vi "Begin.vi"   [LabVIEW 2013]
uses:
  <vilib>/Rock Robotics/SystemInterfaces/DIO/FPGA_DIOPWMChannel.ctl
  <vilib>/Rock Robotics/WPI/SafetyOutput/WPI_SafetyOutputConfigMenu.ctl
  <vilib>/Rock Robotics/SystemInterfaces/DIO/FPGA_DIOChannel.ctl
  <vilib>/Rock Robotics/SystemInterfaces/AI/FPGA_AIGyroChannel.ctl
  <vilib>/Rock Robotics/SystemInterfaces/Typedef/FPGA_TypedefDigitalModule.ctl
  <vilib>/Rock Robotics/WPI/RobotDrive/WPI_RobotDriveOpen4MotorWithJaguar.vi
  <vilib>/Rock Robotics/WPI/Counter/WPI_CounterDigitalInputToDigitalSource.vi
  <vilib>/Rock Robotics/WPI/Counter/WPI_CounterOpen Semi Period Mode.vi
types:
  T1 = typedef "FPGA_DIOChannel.ctl" = enum8{"DIO 1", "DIO 2", "DIO 3", "DIO 4", "DIO 5", "DIO 6", "DIO 7", "DIO 8", "DIO 9", "DIO 10", "DIO 11", "DIO 12", "DIO 13", "DIO 14", "Invalid"}
  T2 = typedef "FPGA_TypedefDigitalModule.ctl" = enum16{"Digital Module 1", "Digital Module 2"}
  T3 = typedef "FPGA_AIGyroChannel.ctl" = enum8{"AI 1", "AI 2", "Invalid"}
  T4 = typedef "WPI_SafetyOutputConfigMenu.ctl" = enum16{"Enable", "Disable"}
  T5 = typedef "FPGA_DIOPWMChannel.ctl" = enum8{"PWM 1", "PWM 2", "PWM 3", "PWM 4", "PWM 5", "PWM 6", "PWM 7", "PWM 8", "PWM 9", "PWM 10", "Invalid"}
  T6 = typedef "WPI_DigitalInputDevRef.ctl" = cluster{"DevStatus":errorcluster, "DIO Channel":T1, "Digital Module":T2}
  T7 = typedef "WPI_RobotDriveDevRef.ctl" = cluster{"DevStatus":errorcluster, "Motors[]":T8[], "Square Inputs":bool, "Max Output":dbl, "Isochronous":bool}
  T8 = typedef "WPI_MotorControlDeviceRef.ctl" = cluster{"DeviceStatus":errorcluster, "Type":enum16{"PWM", "CAN"}, "PWM":cluster{"Digital Module":T2, "PWM Channel":T5, "DeadBand":T9}, "CAN":cluster{"Device Number":u8, "Control Mode":T10, "Semaphore":T11, "Max Vout":dbl}, "Invert":bool, "TransformRef":T12, "InvTransformRef":T12}
  T9 = typedef "WPI_PWMDeadband.ctl" = cluster{"Name":string, "maxPositivePwm":i32, "minPositivePwm":i32, "centerPwm":i32, "maxNegativePwm":i32, "minNegativePwm":i32, "angularRange":u16}
  T10 = typedef "WPI_CANJaguar_ControlMode.ctl" = enum8{"Percent VBus", "Current", "Speed", "Position", "Voltage"}
  T11 = typedef "Semaphore RefNum" = refnum<k1>
  T12 = typedef "WPI_PWMTransform_ConPane.ctl" = refnum<vi>
  T13 = typedef "FPGA_CounterEncoderSourceConvertionLVSourceType.ctl" = cluster{"DevStatus":errorcluster, "AnalogTriggerMode?":bool, "DigitalMode":cluster{"Digital Module":T2, "DIO Channel":T14}, "AnalogTriggerMode":cluster{"AnalogTriggerIndex":T15, "OutputType":T16}}
  T14 = typedef "FPGA_DIODigitalSourceChannel.ctl" = enum8{"DIO 1", "DIO 2", "DIO 3", "DIO 4", "DIO 5", "DIO 6", "DIO 7", "DIO 8", "DIO 9", "DIO 10", "DIO 11", "DIO 12", "DIO 13", "DIO 14", "Disabled"}
  T15 = typedef "FPGA_AnalogTriggerIndex.ctl" = enum8{"Trig 0", "Trig 1", "Trig 2", "Trig 3", "Trig 4", "Trig 5", "Trig 6", "Trig 7", "Invalid"}
  T16 = typedef "FPGA_AnalogTriggerOutType.ctl" = enum16{"InWindow", "TriggerState", "Rising", "Falling"}
  T17 = typedef "WPI_EncoderDevRef.ctl" = cluster{"DevStatus":errorcluster, "EncoderIndex":T18, "CounterIndex":T19, "DistancePerCount":dbl, "Decoding Type":T20}
  T18 = typedef "FPGA_EncoderIdx.ctl" = enum8{"Enc 0", "Enc 1", "Enc 2", "Enc 3", "Invalid"}
  T19 = typedef "FPGA_CounterCtrSystemIndex.ctl" = enum8{"Ctr 0", "Ctr 1", "Ctr 2", "Ctr 3", "Ctr 4", "Ctr 5", "Ctr 6", "Ctr 7", "Invalid"}
  T20 = typedef "WPI_EncoderType.ctl" = enum16{"1x", "2x", "4x"}
  T21 = typedef "WPI_GyroDevRef.ctl" = cluster{"DevStatus":errorcluster, "Analog Module":T22, "Analog Channel":T23, "Offset":dbl, "Gain (VoltsPerDegree/Second)":dbl}
  T22 = typedef "FPGA_TypedefAnalogModule.ctl" = enum16{"Analog Module 1", "Analog Module 2"}
  T23 = typedef "FPGA_AIChannel.ctl" = enum8{"AI 1", "AI 2", "AI 3", "AI 4", "AI 5", "AI 6", "AI 7", "AI 8", "Invalid"}
  T24 = typedef "WPI_CounterDevRef.ctl" = cluster{"DevStatus":errorcluster, "CntIndex":T19}
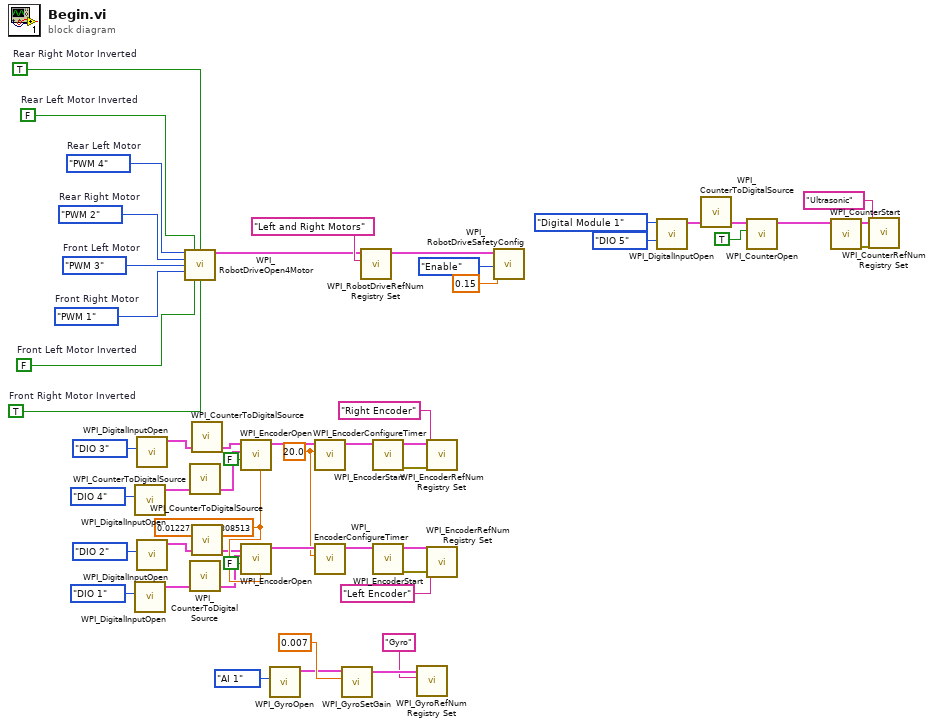
[diagram p0: block diagram]
diagram:
  w44 = 0.01227184630308513 ("DistancePerCount")
  w16 = 20.0 ("Minimum Rate")
  w8 = TRUE  # Front Right Motor Inverted
  w7 = FALSE  # Front Left Motor Inverted
  w6 = TRUE  # Rear Right Motor Inverted
  w5 = FALSE  # Rear Left Motor Inverted
  w4 = FPGA_DIOPWMChannel."PWM 1"  # Front Right Motor
  w3 = FPGA_DIOPWMChannel."PWM 3"  # Front Left Motor
  w2 = FPGA_DIOPWMChannel."PWM 2"  # Rear Right Motor
  w1 = FPGA_DIOPWMChannel."PWM 4"  # Rear Left Motor
  n1 = call <vilib>:"WPI_DigitalInputOpen.vi"("DIO Channel"=FPGA_DIOChannel."DIO 4") -> ("DigitalInputDevRef"=w33:T6)  [unwired: 9 in, 1 out]
  n2 = call <vilib>:"WPI_DigitalInputOpen.vi"("DIO Channel"=FPGA_DIOChannel."DIO 1") -> ("DigitalInputDevRef"=w19:T6)  [unwired: 9 in, 1 out]
  n3 = call <vilib>:"WPI_DigitalInputOpen.vi"("DIO Channel"=FPGA_DIOChannel."DIO 3") -> ("DigitalInputDevRef"=w32:T6)  [unwired: 9 in, 1 out]
  n4 = call <vilib>:"WPI_DigitalInputOpen.vi"("DIO Channel"=FPGA_DIOChannel."DIO 2") -> ("DigitalInputDevRef"=w20:T6)  [unwired: 9 in, 1 out]
  n5 = call-poly <vilib>:"WPI_RobotDriveOpen4Motor.vi"("Rear Left Motor"=w1, "Rear Left Motor Inverted"=w5, "Rear Right Motor Inverted"=w6, "Rear Right Motor"=w2, "Front Left Motor"=w3, "Front Right Motor"=w4, "Front Left Motor Inverted"=w7, "Front Right Motor Inverted"=w8) -> ("RobotDriveDevRef"=w9:T7)  [unwired: 6 in, 1 out]
  n6 = call-poly <vilib>:"WPI_CounterToDigitalSource.vi"("DigitalInputDevRef"=w33) -> ("Digital Source"=w23:T13)  [unwired: 6 in]
  n7 = call-poly <vilib>:"WPI_CounterToDigitalSource.vi"("DigitalInputDevRef"=w19) -> ("Digital Source"=w17:T13)  [unwired: 6 in]
  n8 = call-poly <vilib>:"WPI_CounterToDigitalSource.vi"("DigitalInputDevRef"=w32) -> ("Digital Source"=w36:T13)  [unwired: 6 in]
  n9 = call-poly <vilib>:"WPI_CounterToDigitalSource.vi"("DigitalInputDevRef"=w20) -> ("Digital Source"=w18:T13)  [unwired: 6 in]
  n10 = call <vilib>:"WPI_EncoderOpen.vi"("DistancePerCount"=w44, "Invert Direction (False)"=FALSE, "BSource"=w23, "ASource"=w36) -> ("EncoderDevRef"=w38:T17)  [unwired: 4 in, 3 out]
  n11 = call <vilib>:"WPI_EncoderOpen.vi"("DistancePerCount"=w44, "Invert Direction (False)"=FALSE, "BSource"=w17, "ASource"=w18) -> ("EncoderDevRef"=w34:T17)  [unwired: 4 in, 3 out]
  n12 = call <vilib>:"WPI_GyroOpen.vi"("Analog Channel"=FPGA_AIGyroChannel."AI 1") -> ("GyroDevRef"=w41:T21)  [unwired: 8 in, 2 out]
  n13 = call <vilib>:"WPI_EncoderConfigureTimer.vi"("Minimum Rate"=w16, "EncoderDevRef"=w38) -> ("EncoderDevRef"=w37:T17)  [unwired: 2 in, 7 out]
  n14 = call <vilib>:"WPI_EncoderConfigureTimer.vi"("Minimum Rate"=w16, "EncoderDevRef"=w34) -> ("EncoderDevRef"=w35:T17)  [unwired: 2 in, 7 out]
  n15 = call <vilib>:"WPI_GyroSetGain.vi"("Gain (VoltsPerDegree/Second)"=0.007, "GyroDevRef"=w41) -> ("GyroDevRef"=w43:T21)  [unwired: 8 in, 1 out]
  n16 = call <vilib>:"WPI_RobotDriveRefNum Registry Set.vi"("refnum name"="Left and Right Motors", "RobotDriveDevRef"=w9) -> ("RobotDriveDevRef"=w12:T7)  [unwired: 1 in, 8 out]
  n17 = call <vilib>:"WPI_EncoderStart.vi"("EncoderDevRef"=w37) -> ("error out"=w31:errorcluster, "EncoderDevRef"=w30:T17)  [unwired: 1 in, 8 out]
  n18 = call <vilib>:"WPI_EncoderStart.vi"("EncoderDevRef"=w35) -> ("error out"=w29:errorcluster, "EncoderDevRef"=w28:T17)  [unwired: 1 in, 8 out]
  n19 = call <vilib>:"WPI_GyroRefNum Registry Set.vi"("refnum name"="Gyro", "GyroDevRef"=w43) -> ()  [unwired: 8 in, 2 out]
  n20 = call <vilib>:"WPI_EncoderRefNum Registry Set.vi"("error in (no error)"=w31, "refnum name"="Right Encoder", "EncoderDevRef"=w30) -> ()  [unwired: 7 in, 2 out]
  n21 = call <vilib>:"WPI_EncoderRefNum Registry Set.vi"("error in (no error)"=w29, "refnum name"="Left Encoder", "EncoderDevRef"=w28) -> ()  [unwired: 7 in, 2 out]
  n22 = call <vilib>:"WPI_RobotDriveSafetyConfig.vi"("timeout (s)"=0.15, "mode"=WPI_SafetyOutputConfigMenu."Enable", "RobotDriveDevRef"=w12) -> ()  [unwired: 7 in, 2 out]
  n23 = call <vilib>:"WPI_DigitalInputOpen.vi"("DIO Channel"=FPGA_DIOChannel."DIO 5", "Digital Module (Module 1)"=FPGA_TypedefDigitalModule."Digital Module 1") -> ("DigitalInputDevRef"=w46:T6)  [unwired: 1 in, 8 out]
  n24 = call-poly <vilib>:"WPI_CounterToDigitalSource.vi"("DigitalInputDevRef"=w46) -> ("Digital Source"=w48:T13)  [unwired: 6 in]
  n25 = call-poly <vilib>:"WPI_CounterOpen.vi"("High Pulse (T)"=TRUE, "Source"=w48) -> ("CounterDevRef"=w47:T24)  [unwired: 8 in, 1 out]
  n26 = call <vilib>:"WPI_CounterStart.vi"("CounterDevRef in"=w47) -> ("error out"=w51:errorcluster, "CounterDevRef out"=w52:T24)  [unwired: 9 in]
  n27 = call <vilib>:"WPI_CounterRefNum Registry Set.vi"("error in (no error)"=w51, "refnum name"="Ultrasonic", "CounterDevRef"=w52) -> ()  [unwired: 7 in, 2 out]
